vi "CameraStreamIMAQ.vi"() -> ()   [LabVIEW 2020]
panel:
  out "Image":T1(plugin-control)
  in  "Stop":bool
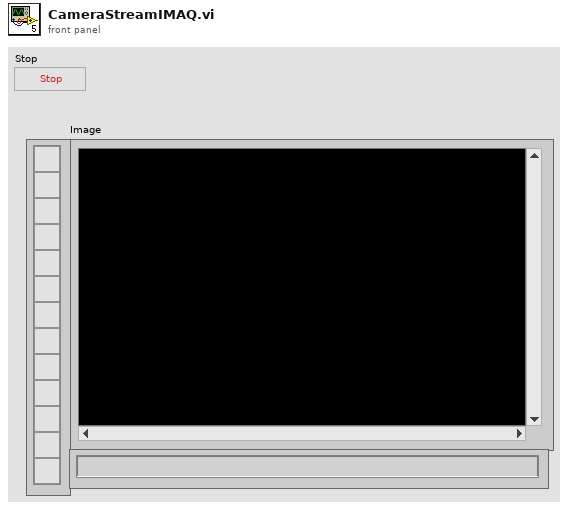
[diagram p1: front panel]
types:
  T1 = typedef "IMAQ Image.ctl" = refnum<image>
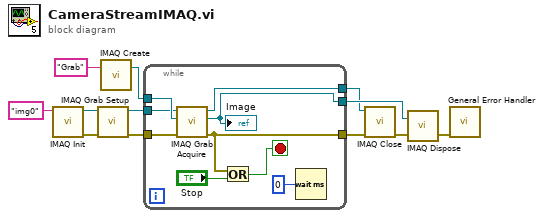
[diagram p0: block diagram]
diagram:
  n1 = call <vilib>:"IMAQ Init.vi"("Interface Name"="img0") -> ("error out"=w10:errorcluster, "IMAQ Session Out"=w12:refnum<k11>)  [unwired: 9 in]
  n2 = call <vilib>:"IMAQ Grab Setup.vi"("error in (no error)"=w10, "IMAQ Session In"=w12) -> ("error out"=w2:errorcluster, "IMAQ Session Out"=w3:refnum<k11>)  [unwired: 8 in]
  n3 = call "IMAQ Create"("Image Name"="Grab") -> ("New Image"=w9:T1)  [unwired: 4 in, 1 out]
  n4 = while {
    tunnel: w2 -> [w14]
    tunnel: w9 -> [w18]
    tunnel: w3 -> [w17]
    tunnel: [w13] -> w7
    tunnel: [w15] -> w8
    tunnel: [w16] -> w6
    stop <- w20 stop-if-true
    n5 = call <vilib>:"IMAQ Grab Acquire.vi"("error in (no error)"=w14, "Image In"=w18, "IMAQ Session In"=w17) -> ("error out"=w13:errorcluster, "Image Out"=w15:T1, "IMAQ Session Out"=w16:refnum<k11>)  [unwired: 5 in, 1 out]
    "Image" <- w15
    n6 = Or(x=w13, y="Stop") -> (x .or. y?=w20:bool)
    n7 = Wait (ms)(milliseconds to wait=u32 0) -> ()  [unwired: 1 out]
  }
  n8 = call <vilib>:"IMAQ Close.vi"("error in (no error)"=w7, "IMAQ Session In"=w6) -> ("error out"=w5:errorcluster)  [unwired: 9 in]
  n9 = call "IMAQ Dispose"("Image"=w8, "error in (no error)"=w5) -> ("error out"=w4:errorcluster)  [unwired: 4 in]
  n10 = call <vilib>:"General Error Handler.vi"("error in (no error)"=w4) -> ()  [unwired: 10 in, 5 out]
